vi "Info2DArray21DClusterArray.vi"(2 "error in (no error)":errorcluster caption="错误输入（无错误）", 3 "2DStringArray":string[][](array[string])=[["121", "23dv"], ["11", "fdfv"], ["33", "bfg"]]) -> (0 "error out":errorcluster caption="错误输出", 1 "1DClusterArray":T1[](array[typedef]))   [LabVIEW 2019]
uses:
  ctl/InfoOfPlayer.ctl
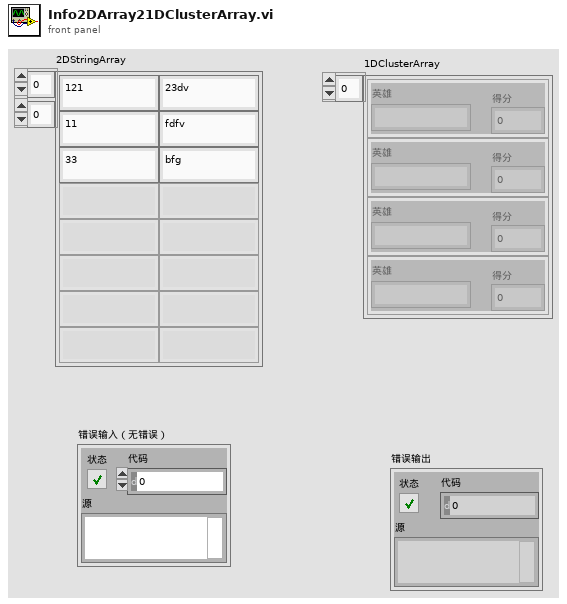
[diagram p1: front panel]
types:
  T1 = typedef "InfoOfPlayer.ctl" = cluster{"得分":i32, "英雄":string}
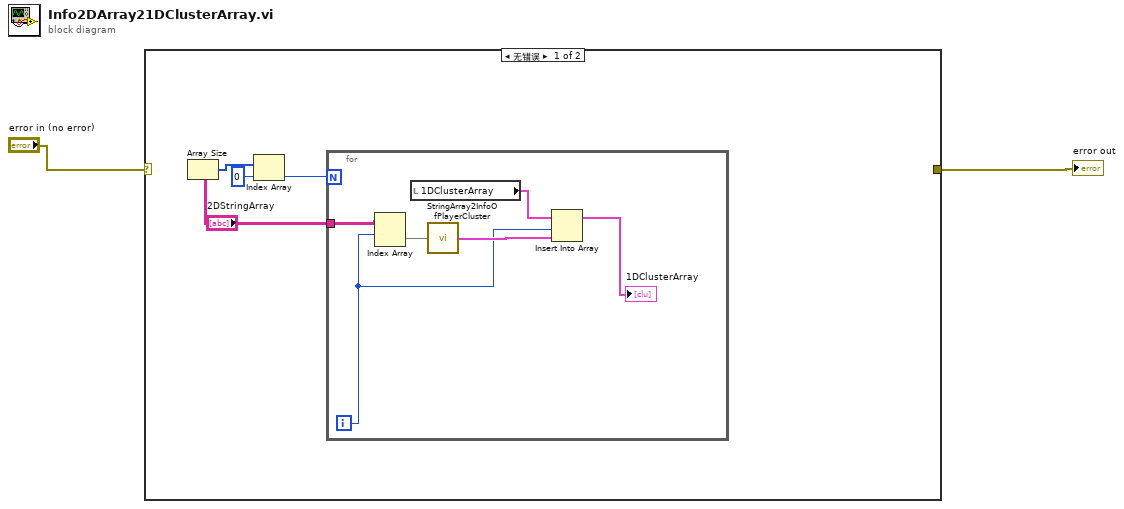
[diagram p0: block diagram]
diagram:
  n1 = case shown="无错误" "error in (no error)" {
    selector: "error in (no error)" -> [_ w13]
    tunnel: [_ w13] -> w1
    frame No Error {
      n2 = Array Size(array="2DStringArray") -> (size(s)=w6:i32[])
      n3 = Index Array(array=w6, index=0 ("索引")) -> (element=w4:i32)
      n4 = for {
        N: w4 -> [_]
        tunnel: "2DStringArray" -> [w12]
        i -> [w9]
        n5 = Index Array(array=w12, index (row)=w9) -> (element=w11:string[])  [unwired: 1 in]
        n6 = local read "1DClusterArray"() -> (w8:T1[])
        n7 = call "StringArray2InfoOfPlayerCluster.vi"("数组"=w11) -> ("玩家信息"=w10:T1)
        n8 = Insert Into Array(array=w8, index=w9, new element=w10) -> (→"1DClusterArray":T1[])
      }
    }
    frame Error {
    }
  }
  "error out" <- w1
